vi "Teleop.vi"(10 "Match Info":T1={"Autonomous Elapsed Seconds"=0.0, "TeleOp Elapsed Seconds"=0.0, "Disabled Elapsed Seconds"=0.0, "Visited Autonomous"=FALSE, "Visited TeleOp"=FALSE, "Visited Disabled"=FALSE, "Autonomous Settings"={"Autonomous Style"=enum."Independent", "VI Refnum"=refnum}}, 11 "Call Context":T2) -> ()   [LabVIEW 2017]
doc: "This VI is called for each TeleOp packet received from the DS where the robot is not disabled. It is often used to read from the joysticks and update I/O or to update setpoints for timed control loops. It should complete and return within 20 milliseconds or it may miss DS packets."
uses:
  Robot Global Data.vi
  <vilib>/Rock Robotics/Network Tables/NT Read String.vi
  <vilib>/Rock Robotics/Network Tables/NT Write Numeric Array.vi
  <vilib>/Rock Robotics/Network Tables/NT Write Boolean Array.vi
  <vilib>/Rock Robotics/Network Tables/NT Read Number.vi
  <vilib>/Rock Robotics/Network Tables/NT Read Boolean.vi
  <vilib>/Rock Robotics/WPI/DriverStation/WPI_DriverStationMatch Info.ctl
  <vilib>/Rock Robotics/WPI/DriverStation/WPI_DriverStationDerivedRobotMode.ctl
panel:
  # "More Changes"
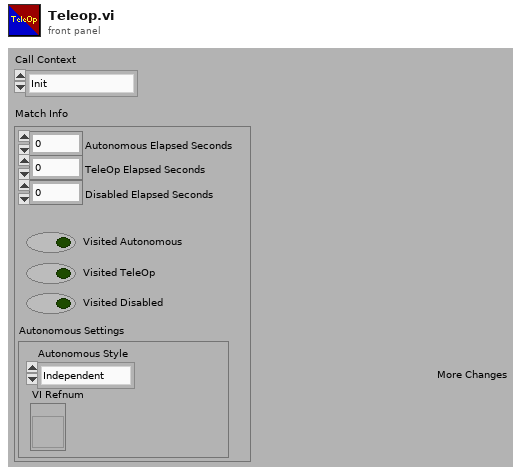
[diagram p1: front panel]
types:
  T1 = typedef "WPI_DriverStationMatch Info.ctl" = cluster{"Autonomous Elapsed Seconds":dbl, "TeleOp Elapsed Seconds":dbl, "Disabled Elapsed Seconds":dbl, "Visited Autonomous":bool, "Visited TeleOp":bool, "Visited Disabled":bool, "Autonomous Settings":cluster{"Autonomous Style":enum16{"Iterative", "Independent"}, "VI Refnum":refnum<vi>}}
  T2 = typedef "WPI_DriverStationDerivedRobotMode.ctl" = enum16{"Init", "Execute", "Stop"}
  T3 = enum16{"1 Xbox Controller", "2 Xbox Controllers"}
  T4 = typedef "TeleopCommands.ctl" = cluster{"Drive Axes":dbl[], "Shooter Forwards":bool, "Shooter Reverse":bool, "Intake Forwards":bool, "Intake Reverse":bool, "Lift Forwards":bool, "Lift Reverse":bool, "Agitator Forwards":bool, "Agitator Reverse":bool, "Left Gear Angle":bool, "Mid Gear Angle":bool, "Right Gear Angle":bool, "Shooter Distance":bool, "Vision Align":bool, "Place Gear":bool, "Command Stop":bool, "Reset Gyro":bool, "Jog Mode?":bool, "Lift Override":bool, "Lift Power":dbl}
  T5 = typedef "WPI_JoystickDevRef.ctl" = cluster{"Device":T6}
  T6 = typedef "WPI_JoystickDeviceEnum.ctl" = enum16{"USB 0", "USB 1", "USB 2", "USB 3", "USB 4", "USB 5"}
  T7 = cluster{"Yaw":dbl, "Roll":dbl, "Pitch":dbl, "Heading":dbl, "Fused Heading":dbl}
  T8 = typedef "WPI_MotorControlDeviceRef.ctl" = cluster{"DeviceStatus":errorcluster, "Type":T9, "PWM":cluster{"PWM Channel":T10, "DeadBand":T11}, "CAN":cluster{"Device Number":u8, "SetOutput VI Ref":variant, "GetOutput VI Ref":variant, "Enable VI Ref":variant, "Disable VI Ref":variant, "Data":variant}, "Invert":bool, "DIO PWM":cluster{"PWM \"Enable\" Channel":T10, "DIOChannel":T12, "PWM Rate":dbl}}
  T9 = typedef "WPI_MotorControlType.ctl" = enum16{"PWM", "CAN", "DIO PWM"}
  T10 = typedef "FPGA_DIOPWMChannel.ctl" = enum8{"PWM 0", "PWM 1", "PWM 2", "PWM 3", "PWM 4", "PWM 5", "PWM 6", "PWM 7", "PWM 8", "PWM 9", "PWM MXP 0", "PWM MXP 1", "PWM MXP 2", "PWM MXP 3", "PWM MXP 4", "PWM MXP 5", "PWM MXP 6", "PWM MXP 7", "PWM MXP 8", "PWM MXP 9", "Invalid"}
  T11 = typedef "WPI_PWMDeadband.ctl" = cluster{"Name":string, "maxPositivePwm":i32, "minPositivePwm":i32, "centerPwm":i32, "maxNegativePwm":i32, "minNegativePwm":i32, "angularRange":u16}
  T12 = typedef "FPGA_DIOChannel.ctl" = enum8{"DIO 0", "DIO 1", "DIO 2", "DIO 3", "DIO 4", "DIO 5", "DIO 6", "DIO 7", "DIO 8", "DIO 9", "DIO MXP 0", "DIO MXP 1", "DIO MXP 2", "DIO MXP 3", "DIO MXP 4", "DIO MXP 5", "DIO MXP 6", "DIO MXP 7", "DIO MXP 8", "DIO MXP 9", "DIO MXP 10", "DIO MXP 11", "DIO MXP 12", "DIO MXP 13", "DIO MXP 14", "DIO MXP 15", "SPI Port CS1", "SPI Port CS2", "SPI Port CS3", "SPI Port MISO", "SPI Port MOSI", "Invalid"}
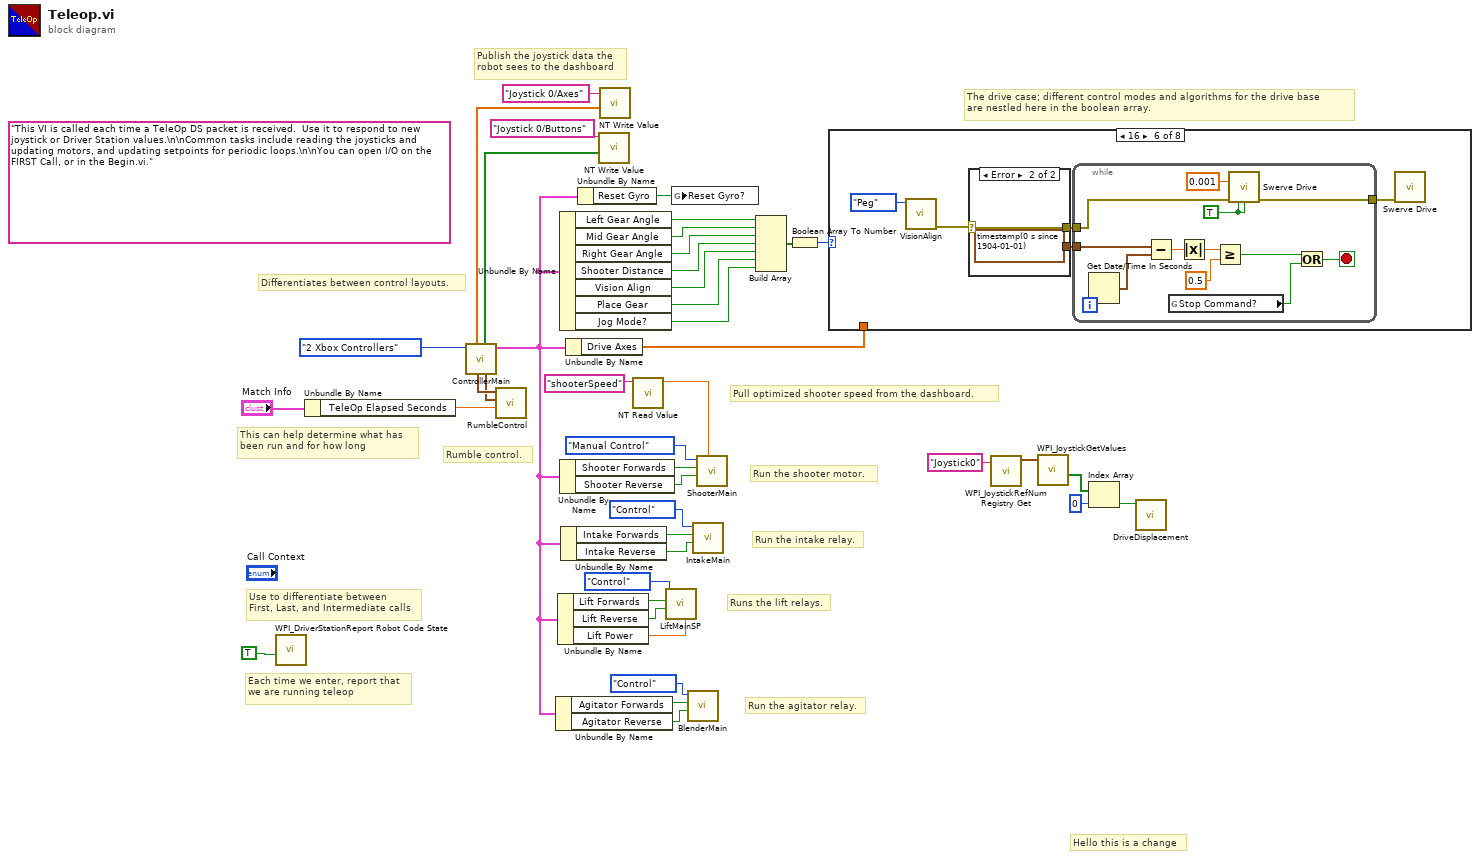
[diagram p0: block diagram]
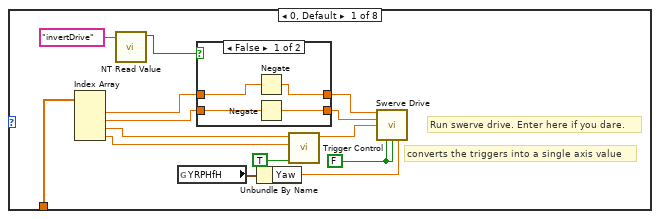
[diagram p2: hidden frame]
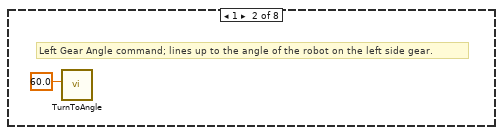
[diagram p4: hidden frame]
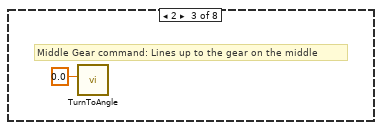
[diagram p5: hidden frame]
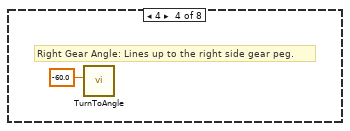
[diagram p6: hidden frame]
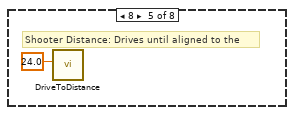
[diagram p7: hidden frame]
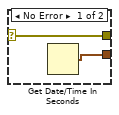
[diagram p8: hidden frame]
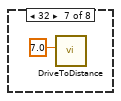
[diagram p9: hidden frame]
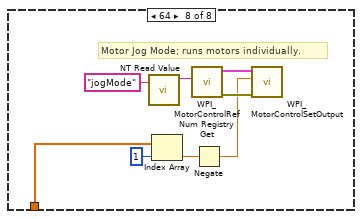
[diagram p10: hidden frame]
diagram:
  (unwired) "This VI is called each time a TeleOp DS packet is received.  Use it to respond to new joystick or Driver Station values.\n\nCommon tasks include reading the joysticks and updating motors, and updating setpoints for periodic loops.\n\nYou can open I/O on the FIRST Call, or in the Begin.vi."
  # "Hello this is a change"
  # "Pull optimized shooter speed from the dashboard."
  # "Runs the lift relays."
  # "The drive case; different control modes and algorithms for the drive base \nare nestled here in the boolean array."
  # "Rumble control."
  # "Differentiates between control layouts."
  # "Run the agitator relay."
  # "Run the intake relay."
  # "Run the shooter motor."
  # "Publish the joystick data the\nrobot sees to the dashboard"
  # "Each time we enter, report that\nwe are running teleop"
  # "Use to differentiate between\nFirst, Last, and Intermediate calls"
  # "This can help determine what has\nbeen run and for how long"
  n1 = call <vilib>:"WPI_DriverStationReport Robot Code State.vi"("TeleOp"=TRUE ("Autonomous")) -> ()  [unwired: 10 in, 1 out]
  n2 = Unbundle By Name("Match Info") -> ("TeleOp Elapsed Seconds"=w21:dbl)
  n3 = call "ControllerMain.vi"("Control Mode"=T3."2 Xbox Controllers") -> ("Robot Inputs"=w19:T4, "Joystick1DevRef"=w22:T5, "Stick0 Buttons"=w35:bool[], "Joystick0DevRef"=w23:T5, "Stick0 Axes"=w36:dbl[])  [unwired: 5 in, 1 out]
  n4 = call "RumbleControl.vi"("Teleop Time"=w21, "JoystickDevRef1"=w22, "JoystickDevRef0"=w23) -> ()  [unwired: 8 in, 1 out]
  n5 = Unbundle By Name(w19) -> ("Agitator Forwards"=w28:bool, "Agitator Reverse"=w26:bool)
  n6 = Unbundle By Name(w19) -> ("Lift Forwards"=w8:bool, "Lift Reverse"=w7:bool, "Lift Power"=w6:dbl)
  n7 = Unbundle By Name(w19) -> ("Left Gear Angle"=w18:bool, "Mid Gear Angle"=w17:bool, "Right Gear Angle"=w16:bool, "Shooter Distance"=w15:bool, "Vision Align"=w14:bool, "Place Gear"=w13:bool, "Jog Mode?"=w11:bool)
  n8 = Unbundle By Name(w19) -> ("Shooter Forwards"=w33:bool, "Shooter Reverse"=w32:bool)
  n9 = Unbundle By Name(w19) -> ("Intake Forwards"=w30:bool, "Intake Reverse"=w29:bool)
  n10 = Unbundle By Name(w19) -> ("Drive Axes"=w38:dbl[])
  n11 = Unbundle By Name(w19) -> ("Reset Gyro"=w12:bool)
  n12 = call-poly <vilib>:"NT Write Value.vi"("Boolean Array"=w35, "Name"="Joystick 0/Buttons") -> ()  [unwired: 9 in, 1 out]
  n13 = call-poly <vilib>:"NT Write Value.vi"("Numeric Array"=w36, "Name"="Joystick 0/Axes") -> ()  [unwired: 9 in, 1 out]
  n14 = call-poly <vilib>:"NT Read Value.vi"("Name"="shooterSpeed") -> ("Numeric"=w10:dbl)  [unwired: 9 in, 1 out]
  n15 = call "LiftMainSP.vi"("Power"=w6, "Reverse"=w7, "Forward"=w8, "Control Mode"=enum16{"Open", "Control"}."Control") -> ()  [unwired: 7 in, 1 out]
  n16 = global write "Robot Global Data.vi" "Reset Gyro?"(w12) -> ()
  n17 = call "BlenderMain.vi"("Reverse"=w26, "Forward"=w28, "Control Mode"=enum16{"Open", "Control"}."Control") -> ()  [unwired: 8 in, 1 out]
  n18 = call "IntakeMain.vi"("Reverse"=w29, "Forward"=w30, "Control Mode"=enum16{"Open", "Control"}."Control") -> ()  [unwired: 6 in, 1 out]
  n19 = call "ShooterMain.vi"("Manual Input"=w10, "Reverse"=w32, "Forward"=w33, "Mode"=enum16{"Open", "PID Control", "Manual Control"}."Manual Control") -> ()  [unwired: 6 in, 2 out]
  n20 = Build Array(w18, w17, w16, w15, w14, w13, w11) -> (w24:bool[])
  n21 = Boolean Array To Number(Boolean array=w24) -> (number=w20:u32)
  n22 = case shown="16" w20 {
    tunnel: w38 -> [w56 _ _ _ _ _ _ w96]
    frame 0, Default {
      w49 = FALSE ("Robot Centric?")
      # "converts the triggers into a single axis value"
      # "Run swerve drive. Enter here if you dare."
      n23 = Index Array(array=w56) -> (element #1=w48:dbl, element #2=w47:dbl, element #3=w55:dbl, element #4=w54:dbl)  [unwired: 4 in]
      n24 = call-poly <vilib>:"NT Read Value.vi"("Name"="invertDrive") -> ("Boolean"=w43:bool)  [unwired: 9 in, 1 out]
      n25 = global read "Robot Global Data.vi" "YRPHfH"() -> (w51:T7)
      n26 = case shown="False" w43 {
        tunnel: w48 -> [w60 w62]
        tunnel: w47 -> [w59 w61]
        tunnel: [w58 w62] -> w46
        tunnel: [w57 w61] -> w45
        frame False {
          n27 = Negate(x=w60) -> (-x=w58:dbl)
          n28 = Negate(x=w59) -> (-x=w57:dbl)
        }
        frame True {
        }
      }
      n29 = Unbundle By Name(w51) -> ("Yaw"=w50:dbl)
      n30 = call "Trigger Control.vi"("Invert?"=TRUE, "Axis 2 In"=w54, "Axis 1 In"=w55) -> ("Axis Out"=w52:dbl)  [unwired: 8 in]
      n31 = call "Swerve Drive.vi"("X"=w46, "Y"=w45, "Z"=w52, "Robot Centric?"=w49, "Autonomous?"=w49, "Yaw"=w50) -> ()  [unwired: 5 in, 5 out]
    }
    frame 1 {
      # "Left Gear Angle command; lines up to the angle of the robot on the left side gear."
      n32 = call "TurnToAngle.vi"("Target Angle"=60.0) -> ()  [unwired: 10 in, 1 out]
    }
    frame 2 {
      # "Middle Gear command: Lines up to the gear on the middle"
      n33 = call "TurnToAngle.vi"("Target Angle"=0.0) -> ()  [unwired: 10 in, 1 out]
    }
    frame 4 {
      # "Right Gear Angle: Lines up to the right side gear peg."
      n34 = call "TurnToAngle.vi"("Target Angle"=-60.0) -> ()  [unwired: 10 in, 1 out]
    }
    frame 8 {
      # "Shooter Distance: Drives until aligned to the"
      n35 = call "DriveToDistance.vi"("Distance"=24.0 ("Setpoint")) -> ()  [unwired: 10 in, 1 out]
    }
    frame 16 {
      n36 = call "VisionAlign.vi"("Control Mode"=enum16{"Boiler", "Peg"}."Peg") -> ("Error Out"=w68:errorcluster)  [unwired: 10 in]
      n37 = case shown="Error" w68 {
        selector: w68 -> [w72 w74]
        tunnel: [w73 timestamp(0 s since 1904-01-01) ("seconds since 1Jan1904")] -> w70
        tunnel: [w72 w74] -> w67
        frame No Error {
          n38 = Get Date/Time In Seconds() -> (seconds since 1Jan1904=w73:timestamp)
        }
        frame Error {
        }
      }
      n39 = while {
        tunnel: w70 -> [w87]
        tunnel: [w80] -> w69
        tunnel: w67 -> [w77]
        stop <- w78 stop-if-true
        w82 = TRUE ("Robot Centric?")
        n40 = Get Date/Time In Seconds() -> (seconds since 1Jan1904=w86:timestamp)
        n41 = Subtract(x=w87, y=w86) -> (x-y=w85:dbl)
        n42 = global read "Robot Global Data.vi" "Stop Command?"() -> (w76:bool)
        n43 = Absolute Value(x=w85) -> (abs(x)=w84:dbl)
        n44 = Greater Or Equal?(x=w84, y=0.5) -> (x >= y?=w79:bool)
        n45 = call "Swerve Drive.vi"("Y"=0.001, "Error In"=w77, "Robot Centric?"=w82, "Autonomous?"=w82) -> ("Error Out"=w80:errorcluster)  [unwired: 7 in, 4 out]
        n46 = Or(x=w79, y=w76) -> (x .or. y?=w78:bool)
      }
      n47 = call "Swerve Drive.vi"("Error In"=w69) -> ()  [unwired: 10 in, 5 out]
    }
    frame 32 {
      n48 = call "DriveToDistance.vi"("Distance"=7.0 ("Setpoint")) -> ()  [unwired: 10 in, 1 out]
    }
    frame 64 {
      # "Motor Jog Mode; runs motors individually."
      n49 = call-poly <vilib>:"NT Read Value.vi"("Name"="jogMode") -> ("String"=w93:string)  [unwired: 9 in, 1 out]
      n50 = Index Array(array=w96, index=1) -> (element=w94:dbl)
      n51 = call <vilib>:"WPI_MotorControlRefNum Registry Get.vi"("refnum name"=w93) -> ("error out"=w92:errorcluster, "MotorControlDevRef"=w91:T8)  [unwired: 9 in]
      n52 = Negate(x=w94) -> (-x=w90:dbl)
      n53 = call <vilib>:"WPI_MotorControlSetOutput.vi"("error in (no error)"=w92, "Output"=w90, "MotorControlDevRef"=w91) -> ()  [unwired: 6 in, 3 out]
    }
  }
  n54 = call <vilib>:"WPI_JoystickRefNum Registry Get.vi"("refnum name"="Joystick0") -> ("JoystickDevRef"=w4:T5)  [unwired: 9 in, 1 out]
  n55 = call <vilib>:"WPI_JoystickGetValues.vi"("JoystickDevRef"=w4) -> ("Buttons"=w3:bool[])  [unwired: 6 in, 4 out]
  n56 = Index Array(array=w3, index=0) -> (element=w1:bool)
  n57 = call "DriveDisplacement.vi"("Boolean"=w1) -> ()  [unwired: 10 in, 1 out]
